vi "HIOKI PW3390 Motor Phase 0Adjust.vi"(0 "VISA Resource":refnum<visa-resource-name>, 5 "Phase 0Adjust (0: SET)":enum16{"SET", "CLEAR"}(ring), 11 "error in (no error)":errorcluster, 12 "OPC query (T: ON)":bool=TRUE, 13 "Error Out (F: Off)":bool) -> (4 "VISA Resource out":refnum<visa-resource-name>, 15 "error out":errorcluster)   [LabVIEW 2009]
doc: "Executes and clears the Motor Analysis Option Phase Zero Adjust.\n\nPhase 0Adjust\n Executes the Phase Zero Adjust for the motor analysis. Phase Zero Adjust is available only when CH B is set for pulse input and [Harm sync src] is set to [Ext]."
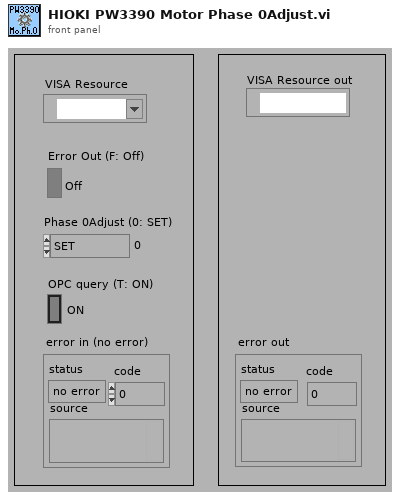
[diagram p1: front panel]
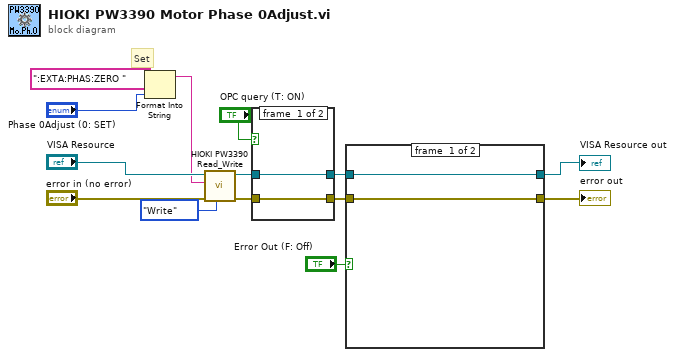
[diagram p0: block diagram]
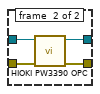
[diagram p2: hidden frame]
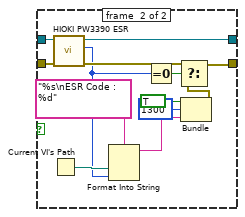
[diagram p3: hidden frame]
diagram:
  # "Set"
  n1 = Format Into String(initial string=":EXTA:PHAS:ZERO ", "Phase 0Adjust (0: SET)") -> (resulting string=w8:string)  [unwired: 2 in, 1 out]
  n2 = call <instrlib>:"HIOKI PW3390 Read_Write.vi"("Read/Write"=enum16{"Read", "Write"}."Write", "error in (no error)"="error in (no error)", "data in"=w8, "VISA Resource"="VISA Resource") -> ("error out"=w3:errorcluster, "VISA Resource out"=w4:refnum<visa-resource-name>)  [unwired: 5 in, 1 out]
  n3 = case shown="TRUE" "OPC query (T: ON)" {
    tunnel: [w16 w20] -> w2
    tunnel: [w15 w19] -> w1
    tunnel: w4 -> [w16 w18]
    tunnel: w3 -> [w15 w17]
    frame #0 {
    }
    frame #1 {
      n4 = call <instrlib>:"HIOKI PW3390 OPC.vi"("error in (no error)"=w17, "VISA Resource"=w18) -> ("error out"=w19:errorcluster, "VISA Resource out"=w20:refnum<visa-resource-name>)  [unwired: 7 in, 1 out]
    }
  }
  n5 = case shown="TRUE" "Error Out (F: Off)" {
    tunnel: w2 -> [w22 w35]
    tunnel: w1 -> [w21 w34]
    tunnel: [w21 w24] -> w11
    tunnel: [w22 w33] -> w6
    frame #0 {
    }
    frame #1 {
      n6 = Current VI's Path() -> (path=w31:path)
      n7 = call <instrlib>:"HIOKI PW3390 ESR.vi"("error in (no error)"=w34, "VISA Resource"=w35) -> ("error out"=w25:errorcluster, "Output Value"=w23:u8, "VISA Resource out"=w33:refnum<visa-resource-name>)  [unwired: 6 in, 1 out]
      n8 = Format Into String(format string="%s\nESR Code : %d", w31, w23) -> (resulting string=w27:string)  [unwired: 2 in, 1 out]
      n9 = Equal To 0?(x=w23) -> (x = 0?=w32:bool)
      n10 = Bundle("status"=TRUE, "code"=1300, w27) -> (w26:cluster{"status":bool, "code":i32, string})  [unwired: 1 in]
      n11 = Select(t=w25, s=w32, f=w26) -> (s? t:f=w24:errorcluster)
    }
  }
  "error out" <- w11
  "VISA Resource out" <- w6
